vi "Reload constants wait time.vi"(8 "millisecond timer value in":u32, 11 "Reload Constants":bool) -> (0 "millisecond timer value out":u32, 3 "Tell Robot to reload constants":bool)   [LabVIEW 2013]
panel:
  in  "Time to send reload to robot":u32=750
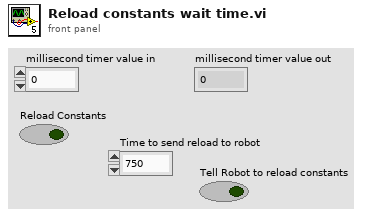
[diagram p1: front panel]
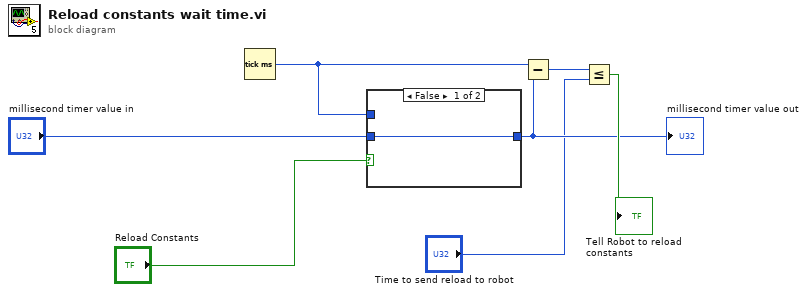
[diagram p0: block diagram]
diagram:
  n1 = Tick Count (ms)() -> (millisecond timer value=w4:u32)
  n2 = case shown="False" "Reload Constants" {
    tunnel: [w8 w9] -> w5
    tunnel: "millisecond timer value in" -> [w8 _]
    tunnel: w4 -> [_ w9]
    frame False {
    }
    frame True {
    }
  }
  "millisecond timer value out" <- w5
  n3 = Subtract(x=w4, y=w5) -> (x-y=w6:u32)
  n4 = Less Or Equal?(x=w6, y="Time to send reload to robot") -> (x <= y?=→"Tell Robot to reload constants":bool)
